vi "λ.vi"(11 "Real Matrix":T1 caption="系数矩阵") -> (3 "λ":dbl)   [LabVIEW 2017]
uses:
  <vilib>/Analysis/Matrix/Datatypes/RealMatrix.ctl
  <vilib>/Analysis/_algsub.llb/Real Matrix Condition Number.vi
  <vilib>/Analysis/Matrix/Numeric/Add/Add - RM,RM.vi
  <vilib>/Analysis/NI_AALPro.lvlib
  <vilib>/Analysis/Matrix/NI_Matrix.lvlib
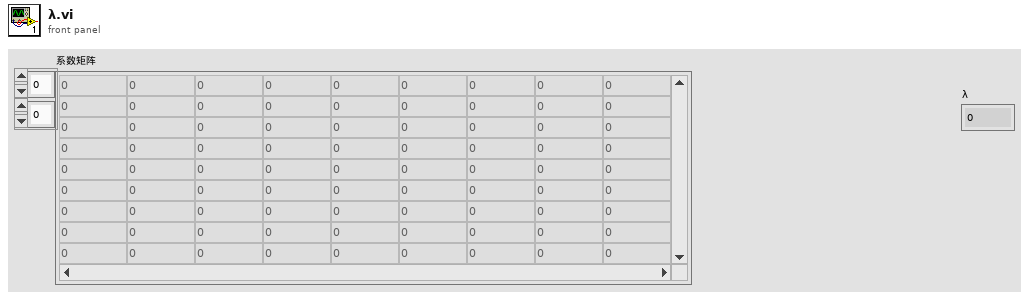
[diagram p1: front panel]
types:
  T1 = typedef "NI_Matrix.lvlib/RealMatrix.ctl" = dbl[][]
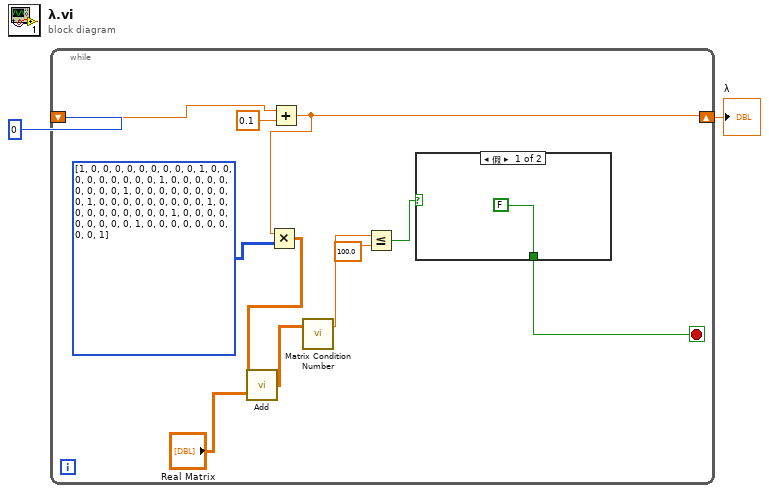
[diagram p0: block diagram]
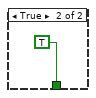
[diagram p2: hidden frame]
diagram:
  n1 = while {
    shift-right: [w5] -> w1
    shift-left: 0 -> [w8]
    stop <- w10 stop-if-true
    n2 = Add(x=w8, y=0.1) -> (x+y=w5:dbl)
    n3 = Multiply(x=w5, y=i32[][] [[1, 0, 0, 0, 0, 0, 0, 0, 0], [0, 1, 0, 0, 0, 0, 0, 0, 0], [0, 0, 1, 0, 0, 0, 0, 0, 0], [0, 0, 0, 1, 0, 0, 0, 0, 0], [0, 0, 0, 0, 1, 0, 0, 0, 0], [0, 0, 0, 0, 0, 1, 0, 0, 0], [0, 0, 0, 0, 0, 0, 1, 0, 0], [0, 0, 0, 0, 0, 0, 0, 1, 0], [0, 0, 0, 0, 0, 0, 0, 0, 1]]) -> (x*y=w4:dbl[][])
    n4 = call-poly <vilib>:"Add.vi"("Real Matrix B"="Real Matrix", "Real Matrix A"=w4) -> ("A + B"=w3:T1)
    n5 = call-poly <vilib>:"Matrix Condition Number.vi"("Input Matrix"=w3) -> ("condition number"=w13:dbl)  [unwired: 1 in, 1 out]
    n6 = Less Or Equal?(x=w13, y=100.0) -> (x <= y?=w11:bool)
    n7 = case shown="假" w11 {
      tunnel: [FALSE TRUE] -> w10
      frame False {
      }
      frame True {
      }
    }
  }
  "λ" <- w1
